vi "Global 1.vi"() -> ()   [LabVIEW 2017]
panel:
  out "IsFinished?":bool=TRUE
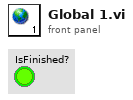
[diagram p1: front panel]
diagram:
